vi "PDE_SpMtrx_Mtrx x Vec.vi"(10 "X":dbl[](array[numeric]), 11 "Sparse Mtrx":T1) -> (3 "Mtrx x X":dbl[](array[numeric]))   [LabVIEW 2017, in "NI_PDE.lvlib"]
uses:
  <vilib>/gmath/NI_PDE.lvlib
  <vilib>/gmath/pde.llb/Common/PDE_Sparse Mtrx.ctl
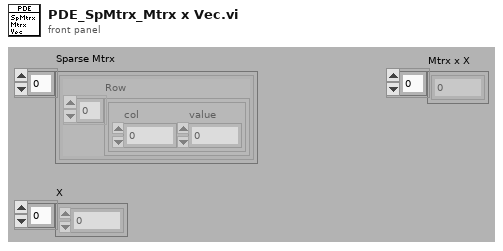
[diagram p1: front panel]
types:
  T1 = typedef "NI_PDE.lvlib/PDE_Sparse Mtrx.ctl" = cluster{"Row":cluster{"col":i32, "value":dbl}[]}[]
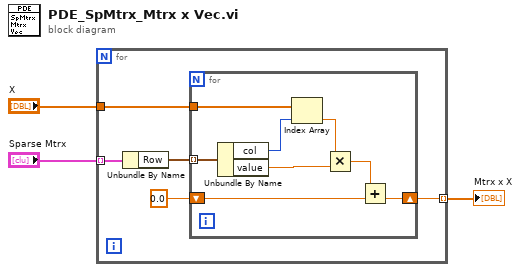
[diagram p0: block diagram]
diagram:
  n1 = for {
    tunnel: "X" -> [w7]
    tunnel: "Sparse Mtrx" -> [w6] mode=indexing
    tunnel: [w4] -> w1 mode=indexing
    n2 = Unbundle By Name(w6) -> ("Row"=w8:cluster{"col":i32, "value":dbl}[])
    n3 = for {
      tunnel: w8 -> [w16] mode=indexing
      tunnel: w7 -> [w15]
      shift-right: [w9] -> w4
      shift-left: 0.0 -> [w10]
      n4 = Unbundle By Name(w16) -> ("col"=w14:i32, "value"=w12:dbl)
      n5 = Index Array(array=w15, index=w14) -> (element=w13:dbl)
      n6 = Multiply(x=w13, y=w12) -> (x*y=w11:dbl)
      n7 = Add(x=w11, y=w10) -> (x+y=w9:dbl)
    }
  }
  "Mtrx x X" <- w1
